vi "Get which board.vi"(8 "error in (no error)":errorcluster, 11 "Assembly Line Input in":refnum<class "Assembly Line Input.lvclass">) -> (0 "error out":errorcluster, 2 "which board":T1, 3 "Assembly Line Input out":refnum<class "Assembly Line Input.lvclass">)   [LabVIEW 2018, in "Assembly Line Input.lvclass"]
uses:
  Assembly Line Input.lvclass
  Common/Board Type Enum.ctl
  Assembly Line Input.lvclass/Assembly Line Input.ctl
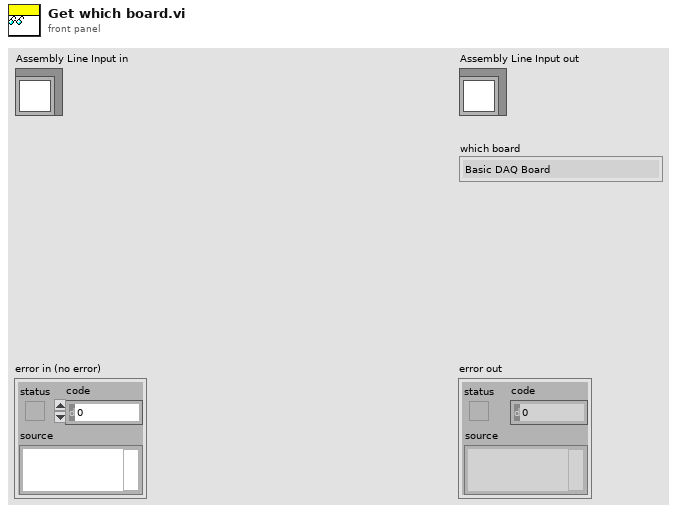
[diagram p1: front panel]
types:
  T1 = typedef "Board Type Enum.ctl" = enum16{"Basic DAQ Board", "Elite DAQ Board", "GPIB Board"}
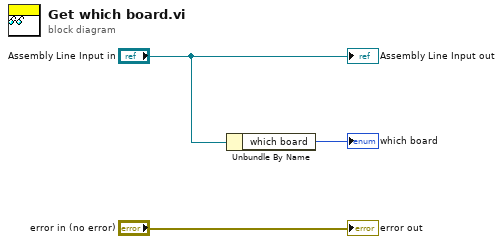
[diagram p0: block diagram]
diagram:
  n1 = Unbundle By Name("Assembly Line Input in") -> ("which board"=→"which board":T1)
  "error out" <- "error in (no error)"
  "Assembly Line Input out" <- "Assembly Line Input in"
